vi "selectRowsOutputManual.vi"(7 "测试类型":string, 8 "error in (no error)":errorcluster, 9 "交流通道":u16(ring) items=["直流CH1", "直流CH2", "直流CH3", "直流CH4", "直流CH5", "直流CH6", "直流CH7", "直流CH8", "交流CH1", "交流CH2"], 10 "直流通道":u16(ring) items=["直流CH1", "直流CH2", "直流CH3", "直流CH4", "直流CH5", "直流CH6", "直流CH7", "直流CH8"], 11 "数据类型":u16(ring) items=["直流", "交流"]) -> (0 "error out 2":errorcluster, 3 "data":string[][](array[string]))   [LabVIEW 2014]
uses:
  <vilib>/addons/database/Connection.llb/DB Tools Open Connec (String).vi
  <vilib>/addons/database/Connection.llb/Conn Execute.vi
  <vilib>/addons/database/Recordset.llb/Rec Fetch Recordset Data (R).vi
  <vilib>/addons/database/Recordset.llb/Rec Destroy - Connection.vi
  <vilib>/addons/database/_DB Variant To Data/Database Variant To Data.xnode
  <vilib>/addons/database/NI_Database_API.lvlib
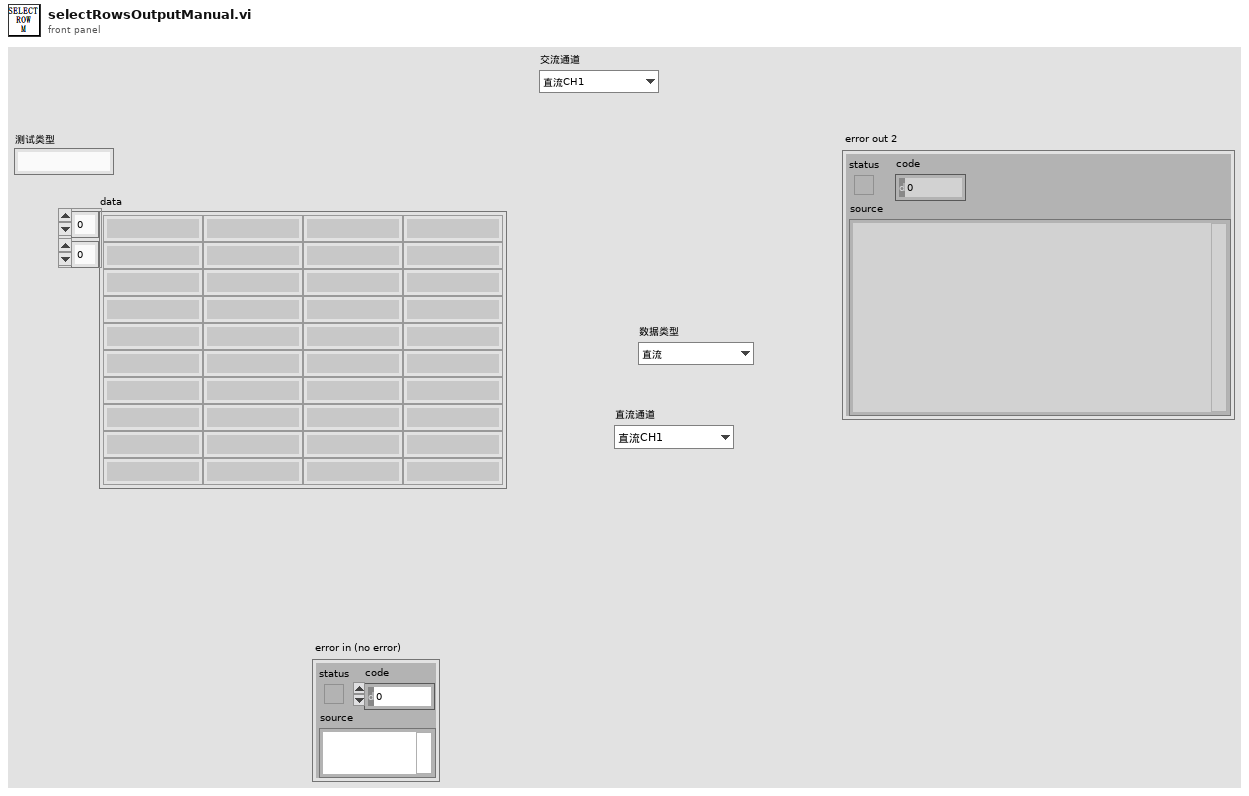
[diagram p1: front panel]
types:
  T1 = typedef "NI_Database_API.lvlib/Conn ObjectReference.ctl" = refnum<k1>
  T2 = typedef "NI_Database_API.lvlib/Rec ObjectReference.ctl" = refnum<k1>
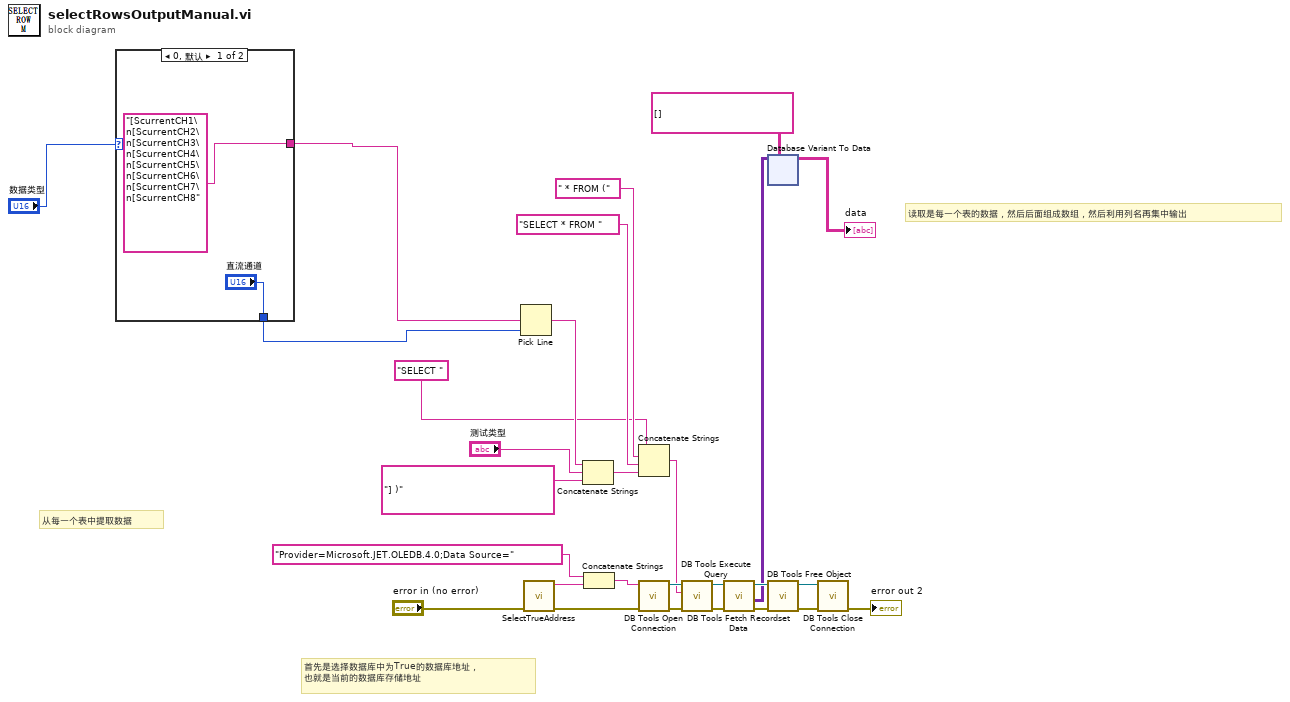
[diagram p0: block diagram]
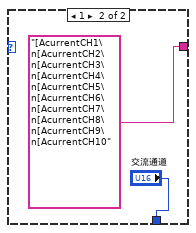
[diagram p2: hidden frame]
diagram:
  # "从每一个表中提取数据"
  # "读取是每一个表的数据，然后后面组成数组，然后利用列名再集中输出"
  # "首先是选择数据库中为True的数据库地址，\n也就是当前的数据库存储地址"
  n1 = case shown="0, 默认" "数据类型" {
    tunnel: ["[ScurrentCH1\n[ScurrentCH2\n[ScurrentCH3\n[ScurrentCH4\n[ScurrentCH5\n[ScurrentCH6\n[ScurrentCH7\n[ScurrentCH8" ("多行字符串") "[AcurrentCH1\n[AcurrentCH2\n[AcurrentCH3\n[AcurrentCH4\n[AcurrentCH5\n[AcurrentCH6\n[AcurrentCH7\n[AcurrentCH8\n[AcurrentCH9\n[AcurrentCH10"] -> w27
    tunnel: ["直流通道" "交流通道"] -> w28
    frame 0, Default {
    }
    frame 1 {
    }
  }
  n2 = Pick Line(multi-line string=w27, line index=w28) -> (output string=w4:string)  [unwired: 1 in]
  n3 = call "SelectTrueAddress.vi"("error in (no error)"="error in (no error)") -> ("error out"=w10:errorcluster, "元素"=w12:string)  [unwired: 9 in]
  n4 = Concatenate Strings(w4, "测试类型", "] )") -> (w22:string)
  n5 = Concatenate Strings("Provider=Microsoft.JET.OLEDB.4.0;Data Source=", w12) -> (w11:string)
  n6 = Concatenate Strings("SELECT ", " * FROM (" ("字符串"), "SELECT * FROM ", w22) -> (w7:string)
  n7 = call-poly <vilib>:"DB Tools Open Connection.vi"("error in (no error)"=w10, "connection information"=w11) -> ("error out"=w8:errorcluster, "connection reference"=w9:T1)  [unwired: 6 in]
  n8 = call-poly <vilib>:"DB Tools Execute Query.vi"("error in (no error)"=w8, "SQL query"=w7, "connection reference"=w9) -> ("error out"=w17:errorcluster, "recordset reference"=w18:T2)  [unwired: 5 in]
  n9 = call-poly <vilib>:"DB Tools Fetch Recordset Data.vi"("error in (no error)"=w17, "recordset reference"=w18) -> ("error out"=w15:errorcluster, "recordset data"=w6:variant[][], "recordset reference out"=w16:T2)  [unwired: 3 in]
  n10 = xnode "Database Variant To Data"("database variant"=w6, "type"=string[][] []) -> ("data"=→"data":string[][])  [unwired: 1 in, 1 out]
  n11 = call-poly <vilib>:"DB Tools Free Object.vi"("error in (no error)"=w15, "recordset reference"=w16) -> ("error out"=w20:errorcluster, "connection reference"=w19:T1)  [unwired: 8 in]
  n12 = call <vilib>:"DB Tools Close Connection.vi"("error in (no error)"=w20, "connection reference"=w19) -> ("error out"=→"error out 2":errorcluster)  [unwired: 5 in]
